vi "convert string to hex.vi"(1 "string":string) -> (0 "hex":u32 format="%.0x")   [LabVIEW 2021, in "TSC Material Theme.lvlib"]
doc: "convert an ARGB text string to the equivalent hex value\n\n<b>Code Developed By:</b>\nTechnology Service Corporation\nwww.tsc.com/atcs\n\nDeveloper:\nDaniel Coons"
uses:
  TSC Material Theme.lvlib
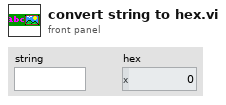
[diagram p1: front panel]
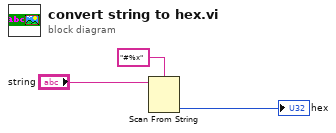
[diagram p0: block diagram]
diagram:
  n1 = Scan From String(format string="#%x", input string="string") -> (output 1=→"hex":u32)  [unwired: 3 in, 3 out]
